vi "dfd_Group Delay_Add Band2.vi"(6 "grid length":dbl, 8 "weight (in)":dbl[](array[numeric]), 9 "d (in)":dbl[](array[numeric]), 10 "freq grid (in)":dbl[](array[numeric]), 11 "Allpass_Band Spec":T1[](array[typedef]) {"subband specs"."weight" format="%.2f"}) -> (0 "weight  (out)":dbl[](array[numeric]), 1 "d  (out)":dbl[](array[numeric]), 2 "freq grid (out)":dbl[](array[numeric]), 3 "Allpass_Band Spec (dup)":T1[](array[typedef]) {"subband specs"."weight" format="%.2f"})   [LabVIEW 2017, in "NI_DigFilter_Design.lvlib"]
uses:
  <vilib>/addons/Digital Filter Design/NI_DigFilter_Design.lvlib
  <vilib>/addons/Digital Filter Design/_GroupDelay.llb/dfd_Group Delay_Band Spec.ctl
  <vilib>/addons/Digital Filter Design/NI_DigFilterLicensed.lvlib
panel:
  # "freq"
  # "group delay"
  # "weight"
  # "freq"
  # "group delay"
  # "weight"
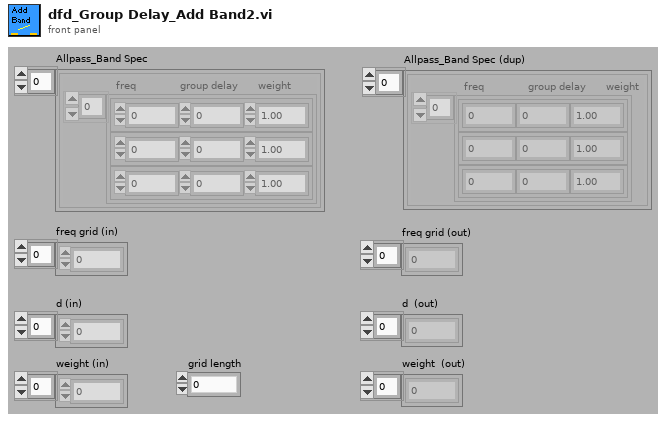
[diagram p1: front panel]
types:
  T1 = typedef "NI_DigFilterLicensed.lvlib/dfd_Group Delay_Band Spec.ctl" = cluster{"subband specs":cluster{"freq":dbl, "group delay":dbl, "weight":dbl}[]}
  T2 = cluster{"freq":dbl, "group delay":dbl, "weight":dbl}[]
  T3 = cluster{"freq":dbl, "group delay":dbl, "weight":dbl}
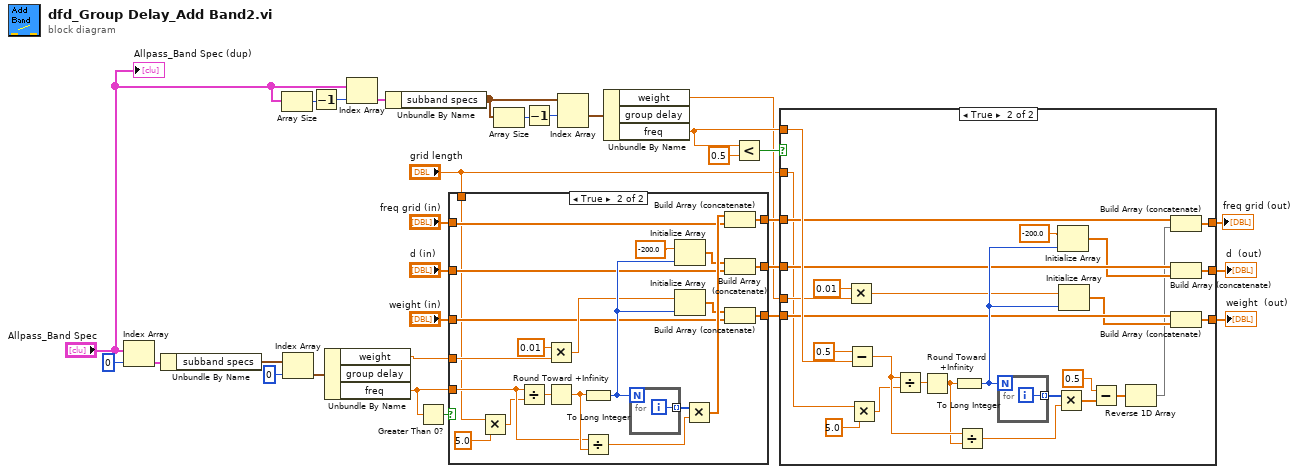
[diagram p0: block diagram]
diagram:
  n1 = Index Array(array="Allpass_Band Spec", index=0) -> (element=w27:T1)
  n2 = Unbundle By Name(w27) -> ("subband specs"=w29:T2)
  n3 = Array Size(array="Allpass_Band Spec") -> (size(s)=w19:i32)
  n4 = Index Array(array=w29, index=0) -> (element=w26:T3)
  n5 = Decrement(x=w19) -> (x-1=w18:i32)
  n6 = Unbundle By Name(w26) -> ("weight"=w20:dbl, "freq"=w21:dbl)  [unwired: 1 out]
  n7 = Index Array(array="Allpass_Band Spec", index=w18) -> (element=w14:T1)
  n8 = Unbundle By Name(w14) -> ("subband specs"=w17:T2)
  n9 = Greater Than 0?(x=w21) -> (x > 0?=w22:bool)
  n10 = case shown="True" w22 {
    tunnel: "freq grid (in)" -> [w33 w38]
    tunnel: "d (in)" -> [w32 w42]
    tunnel: "weight (in)" -> [w31 w40]
    tunnel: [w33 w50] -> w9
    tunnel: [w32 w41] -> w8
    tunnel: [w31 w39] -> w7
    tunnel: w21 -> [_ w37]
    tunnel: w20 -> [_ w46]
    tunnel: "grid length" -> [_ w34]
    frame False {
    }
    frame True {
      n11 = Multiply(x=w34, y=5.0) -> (x*y=w36:dbl)
      n12 = Divide(x=w37, y=w36) -> (x/y=w55:dbl)
      n13 = Multiply(x=0.01, y=w46) -> (x*y=w44:dbl)
      n14 = Round Toward +Infinity(x=w55) -> (ceil(x): smallest int >= x=w54:dbl)
      n15 = To Long Integer(number=w54) -> (32bit integer=w47:i32)
      n16 = Divide(x=w37, y=w54) -> (x/y=w52:dbl)
      n17 = for {
        N: w47 -> [_]
        tunnel: [w56] -> w53 mode=indexing
        i -> [w56]
      }
      n18 = Initialize Array(-200.0 ("element"), w47) -> (w48:dbl[])
      n19 = Initialize Array(w44, w47) -> (w43:dbl[])
      n20 = Multiply(x=w53, y=w52) -> (x*y=w51:dbl[])
      n21 = Build Array (concatenate)(w51, w38) -> (w50:dbl[])
      n22 = Build Array (concatenate)(w48, w42) -> (w41:dbl[])
      n23 = Build Array (concatenate)(w43, w40) -> (w39:dbl[])
    }
  }
  n24 = Array Size(array=w17) -> (size(s)=w12:i32)
  n25 = Decrement(x=w12) -> (x-1=w13:i32)
  n26 = Index Array(array=w17, index #1=w13) -> (element #1=w15:T3)  [unwired: 1 in, 1 out]
  n27 = Unbundle By Name(w15) -> ("weight"=w5:dbl, "freq"=w6:dbl)  [unwired: 1 out]
  n28 = Less?(x=w6, y=0.5) -> (x < y?=w10:bool)
  n29 = case shown="True" w10 {
    tunnel: w9 -> [w59 w76]
    tunnel: w8 -> [w58 w71]
    tunnel: w7 -> [w57 w70]
    tunnel: [w59 w74] -> w4
    tunnel: [w58 w73] -> w3
    tunnel: [w57 w72] -> w2
    tunnel: w6 -> [_ w79]
    tunnel: w5 -> [_ w68]
    tunnel: "grid length" -> [_ w60]
    frame False {
    }
    frame True {
      n30 = Multiply(x=0.01, y=w68) -> (x*y=w66:dbl)
      n31 = Subtract(x=0.5, y=w79) -> (x-y=w84:dbl)
      n32 = Multiply(x=w60, y=5.0) -> (x*y=w62:dbl)
      n33 = Divide(x=w84, y=w62) -> (x/y=w85:dbl)
      n34 = Round Toward +Infinity(x=w85) -> (ceil(x): smallest int >= x=w83:dbl)
      n35 = To Long Integer(number=w83) -> (32bit integer=w77:i32)
      n36 = Divide(x=w84, y=w83) -> (x/y=w81:dbl)
      n37 = for {
        N: w77 -> [_]
        tunnel: [w87] -> w82 mode=indexing
        i -> [w87]
      }
      n38 = Multiply(x=w82, y=w81) -> (x*y=w80:dbl[])
      n39 = Initialize Array(-200.0 ("element"), w77) -> (w69:dbl[])
      n40 = Initialize Array(w66, w77) -> (w65:dbl[])
      n41 = Subtract(x=0.5, y=w80) -> (x-y=w75:dbl[])
      n42 = Reverse 1D Array(array=w75) -> (reversed array=w63:dbl[])
      n43 = Build Array (concatenate)(w76, w63) -> (w74:dbl[])
      n44 = Build Array (concatenate)(w71, w69) -> (w73:dbl[])
      n45 = Build Array (concatenate)(w70, w65) -> (w72:dbl[])
    }
  }
  "freq grid (out)" <- w4
  "weight  (out)" <- w2
  "d  (out)" <- w3
  "Allpass_Band Spec (dup)" <- "Allpass_Band Spec"
